vi "tcp_write_carriers.vi"(5 "Modulation info":T7={"Fs full"=0.0, "Fs high"=0.0, "Fs low"=0.0, "Read size"=5000, "FFT size low"=5000, "df low"=5000.0, "High carriers"=[], "Low carriers"=[], "Hi channels at low"=[7]} {"Hi channels at low" min=0 step=1; "Low carriers" format="%#_6p"; "High carriers" format="%#_6p"}, 7 "ilemt_config":T1={"IO params"={"Conversion"={"Rate"=0.0, "Num cards"=0, "Out channels"=4}, "Carriers"={"Phase shift"=180.0, "Levels"=[[0.8, 0.8, 0.8], [0.03, 0.03, 0.03]], "Delay samples"=73.15}, "TCP"={"Host"="192.168.1.15", "Port"=6666, "Buffering"=6, "Timeout"=6}, "Input channel sign"=[1, 1, 1]}, "High rate STFT"={"Win param"=0.0, "Window type"=0, "Win order"=0, "DFT size"=0, "Channels"=[], "Oversample"=0}, "Low rate STFT"={"Win param"=0.0, "Window type"=0, "Win order"=0, "DFT size"=0, "Channels"=[], "Oversample"=0}, "Filtering "=[]} {"Filtering"."Distortion"."Limit" format="%#_3p"; "Filtering"."Distortion"."LF cut" format="%#_3p"; "Filtering"."Kalman"."Measure noise" format="%#_3p"; "Filtering"."Kalman"."Process noise" format="%#_3p"; "Filtering"."Hum"."Limit" format="%#_3p"; "Filtering"."Hum"."Frequency" format="%#_4p"; "Low rate STFT"."Oversample" min=1 step=1; "Low rate STFT"."Channels" min=0 step=1; "Low rate STFT"."DFT size" min=1 step=1; "Low rate STFT"."Window type" items=["Rectangle"=0, "Hanning"=1, "Hamming"=2, "Blackman-Harris"=3, "Exact Blackman"=4, "Blackman"=5, "Flat Top"=6, "4 Term B-Harris "=7, "7 Term B-Harris"=8, "Low Sidelobe"=9, "Blackman Nuttall"=11, "Triangle"=30, "Bartlett-Hanning"=31, "Bohman"=32, "Parzen"=33, "Welch"=34, "Kaiser"=60, "Dolph-Chebyshev"=61, "Gaussian"=62]; "High rate STFT"."Oversample" min=1 step=1; "High rate STFT"."Channels" min=0 step=1; "High rate STFT"."DFT size" min=1 step=1; "High rate STFT"."Window type" items=["Rectangle"=0, "Hanning"=1, "Hamming"=2, "Blackman-Harris"=3, "Exact Blackman"=4, "Blackman"=5, "Flat Top"=6, "4 Term B-Harris "=7, "7 Term B-Harris"=8, "Low Sidelobe"=9, "Blackman Nuttall"=11, "Triangle"=30, "Bartlett-Hanning"=31, "Bohman"=32, "Parzen"=33, "Welch"=34, "Kaiser"=60, "Dolph-Chebyshev"=61, "Gaussian"=62]; "IO params"."Input channel sign" min=-1 max=1 step=1; "IO params"."Carriers"."Levels" min=0.0 step=0.1; "IO params"."Conversion"."Rate" format="%#_8g"}, 8 "Sequence":u32=3 min=1 max=12, 9 "Carrier output":i32[][](array[numeric]), 11 "Connection in":refnum<k5>) -> (0 "Restart IO":bool, 3 "Connection out":refnum<k5>)   [LabVIEW 2026]
uses:
  processing/modulation_info.ctl
  processing/ilemt_config.ctl
  IO_params.ctl
  processing/stft_params.ctl
  <vilib>/Analysis/4window.llb/windowTd.ctl
  processing/filter_params.ctl
  processing/detrend_mode.ctl
  <vilib>/Analysis/NI_AALPro.lvlib
panel:
  out "Write error":errorcluster
  out "bytes written":i32
  out "Out buffer":i32[](array[numeric])
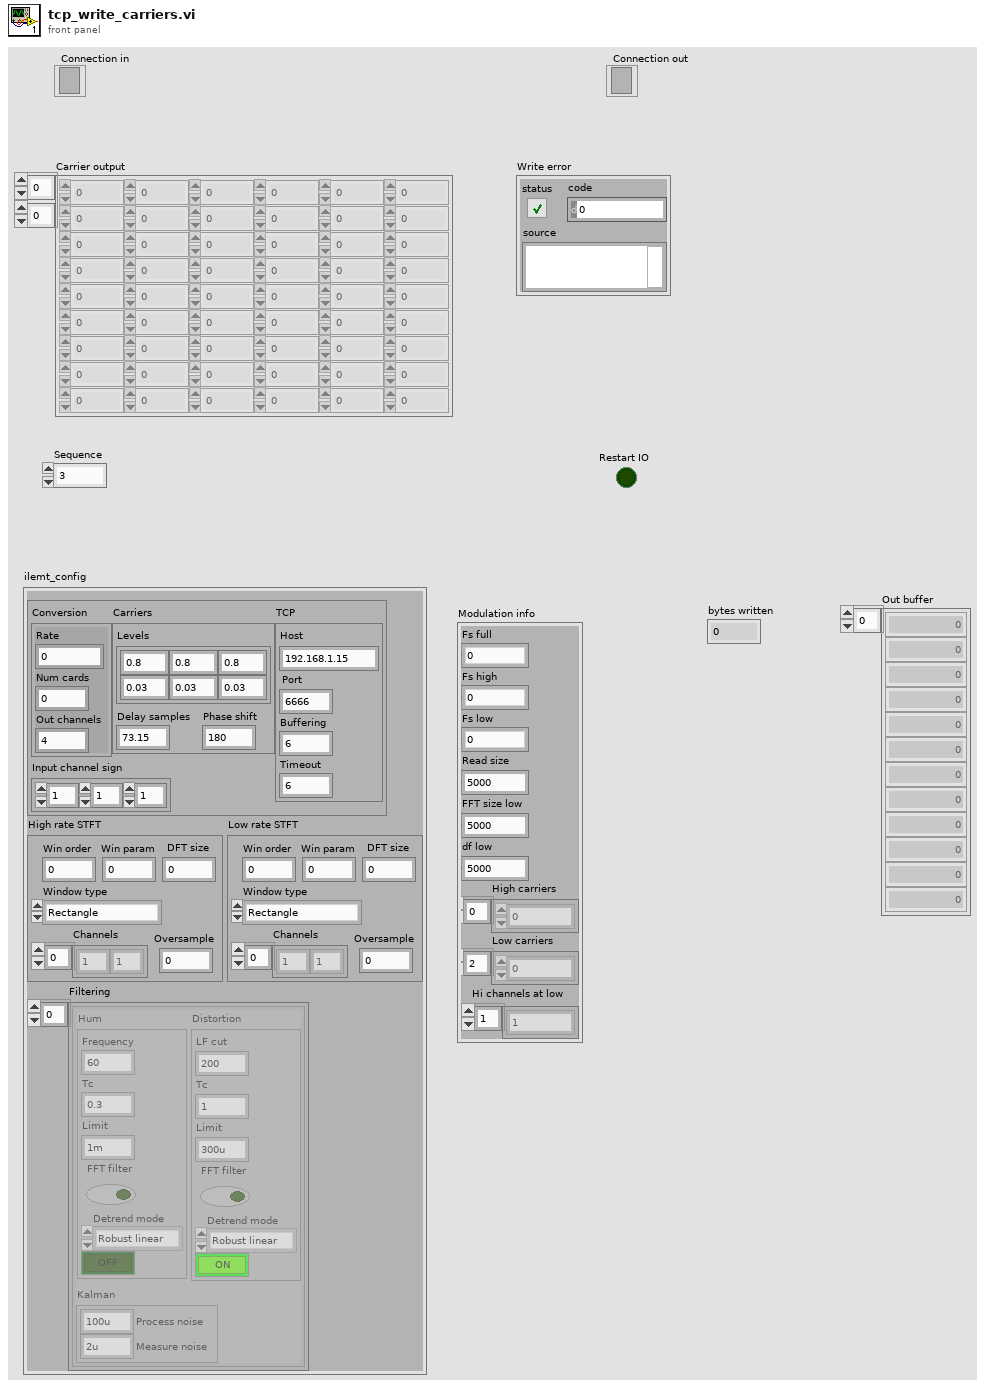
[diagram p1: front panel]
types:
  T1 = typedef "ilemt_config.ctl" = cluster{"IO params":T2, "High rate STFT":T3, "Low rate STFT":T3, "Filtering ":T5[]}
  T2 = typedef "IO_params.ctl" = cluster{"Conversion":cluster{"Rate":dbl, "Num cards":u32, "Out channels":u32}, "Carriers":cluster{"Phase shift":dbl, "Levels":dbl[][], "Delay samples":dbl}, "TCP":cluster{"Host":string, "Port":i32, "Buffering":u32, "Timeout":u32}, "Input channel sign":i32[]}
  T3 = typedef "stft_params.ctl" = cluster{"Win param":dbl, "Window type":T4, "Win order":i32, "DFT size":i32, "Channels":i32[], "Oversample":i32}
  T4 = typedef "NI_AALPro.lvlib/windowTd.ctl" = u32
  T5 = typedef "filter_params.ctl" = cluster{"Hum":cluster{"Frequency":dbl, "Tc":dbl, "Limit":dbl, "FFT filter":bool, "Detrend mode":T6, "Enable":bool}, "Kalman":cluster{"Process noise":dbl, "Measure noise":dbl}, "Distortion":cluster{"LF cut":dbl, "Tc":dbl, "Limit":dbl, "FFT filter":bool, "Detrend mode":T6, "Enable":bool}}
  T6 = typedef "detrend_mode.ctl" = enum16{"Zero mean", "Linear", "Robust linear"}
  T7 = typedef "modulation_info.ctl" = cluster{"Fs full":dbl, "Fs high":dbl, "Fs low":dbl, "Read size":i32, "FFT size low":i32, "df low":dbl, "High carriers":dbl[], "Low carriers":dbl[], "Hi channels at low":i32[]}
  T8 = enum16{"big-endian, network order", "native, host order", "little-endian"}
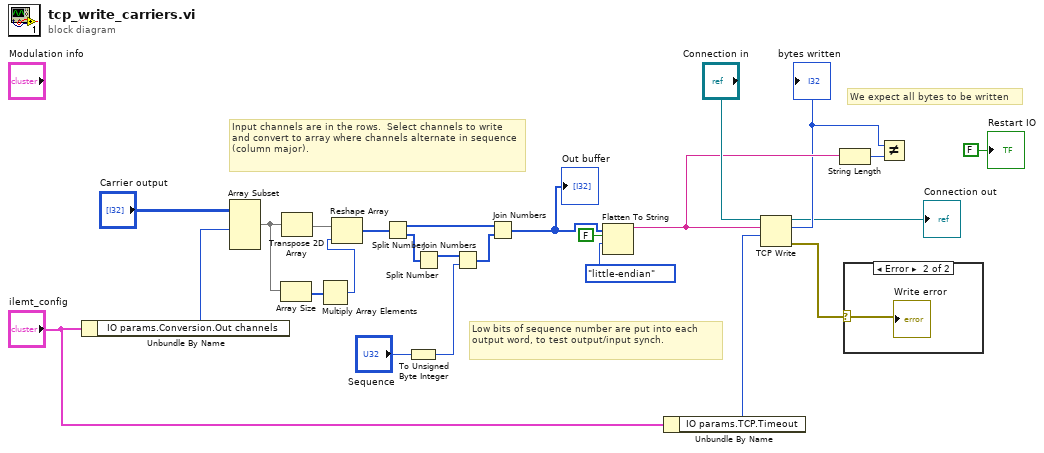
[diagram p0: block diagram]
diagram:
  # "We expect all bytes to be written"
  # "Low bits of sequence number are put into each output word, to test output/input synch."
  # "Input channels are in the rows.  Select channels to write and convert to array where channels alternate in sequence (column major)."
  n1 = Unbundle By Name("ilemt_config") -> ("IO params.Conversion.Out channels"=w8:u32)
  n2 = Array Subset(array="Carrier output", length (row)=w8) -> (w21:i32[][])  [unwired: 3 in]
  n3 = Array Size(array=w21) -> (size(s)=w20:i32[])
  n4 = Transpose 2D Array(2D array=w21) -> (transposed array=w22:i32[][])
  n5 = Multiply Array Elements(1:w20) -> (0:w19:i32)
  n6 = Reshape Array(w22, w19) -> (w18:i32[])
  n7 = Split Number(x=w18) -> (hi(x)=w15:u16[], lo(x)=w17:u16[])
  n8 = To Unsigned Byte Integer(number="Sequence") -> (unsigned 8bit integer=w12:u8)
  n9 = Split Number(x=w17) -> (hi(x)=w13:u8[])  [unwired: 1 out]
  n10 = Join Numbers(hi=w13, lo=w12) -> ((hi.lo)=w14:u16[])
  n11 = Join Numbers(hi=w15, lo=w14) -> ((hi.lo)=w11:u32[])
  "Out buffer" <- w11
  n12 = Flatten To String(anything=w11, prepend array or string size? (T)=FALSE, byte order (0:big-endian, network order)=T8."little-endian") -> (data string=w7:string)  [unwired: 1 in, 2 out]
  n13 = Unbundle By Name("ilemt_config") -> ("IO params.TCP.Timeout"=w3:u32)
  n14 = TCP Write(connection ID="Connection in", data in=w7, 9:w3) -> (connection ID out=→"Connection out":refnum<k5>, bytes written=w6:i32, error out=w9:errorcluster)  [unwired: 1 in]
  "bytes written" <- w6
  n15 = String Length(string=w7) -> (length=w5:i32)
  n16 = case shown="Error" w9 {
    selector: w9 -> [_ w26]
    frame No Error {
    }
    frame Error {
      "Write error" <- w26
    }
  }
  n17 = Not Equal?(x=w6, y=w5) -> ()  [unwired: 1 out]
  "Restart IO" <- FALSE ("Restart IO")
